vi "WriteVisOptionsToINIFile.vi"(7 "section (optional)":string="Logging and Visualization", 8 "error in (no error)":errorcluster, 10 "Visualization Options":T1={"PauseAtStartup"=TRUE, "LogData"=FALSE, "LaunchInSubPanel"=TRUE, "FPMonitor"=0, "FPWindowBounds"={"Left"=0, "Top"=0, "Right"=0, "Bottom"=0}, "MonitorBounds"={"Left"=0, "Top"=0, "Right"=0, "Bottom"=0}, "MeasIndices"=[]}, 11 "INIFilePath":path) -> (0 "error out":errorcluster, 3 "INI File Path out":path)   [LabVIEW 2018, in "Visualization.lvlib" / "VisualizeBase.lvclass"]
uses:
  VisualizeBase.lvclass
  VisualizationOptions.ctl
  <vilib>/Utility/miscctls.llb/LVRectTypeDef.ctl
  <vilib>/Utility/config.llb/NI_LVConfig.lvlib
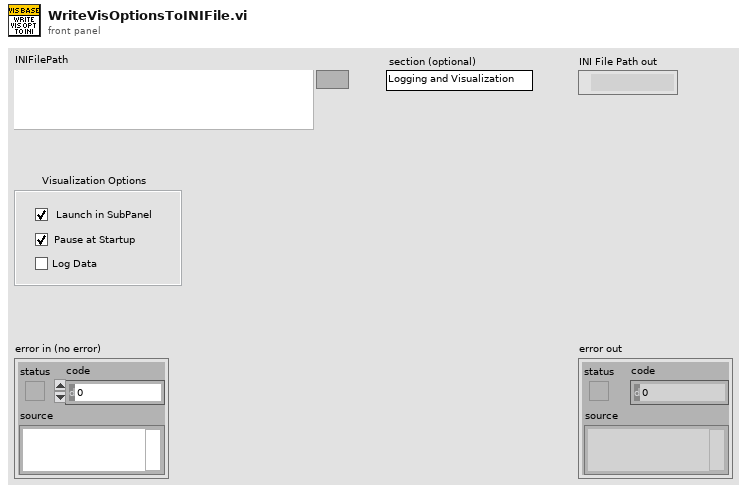
[diagram p1: front panel]
types:
  T1 = typedef "Visualization.lvlib/VisualizeBase.lvclass/VisualizationOptions.ctl" = cluster{"PauseAtStartup":bool, "LogData":bool, "LaunchInSubPanel":bool, "FPMonitor":u16, "FPWindowBounds":T2, "MonitorBounds":cluster{"Left":i16, "Top":i16, "Right":i16, "Bottom":i16}, "MeasIndices":i32[]}
  T2 = typedef "LVRectTypeDef.ctl" = cluster{"Left":i16, "Top":i16, "Right":i16, "Bottom":i16}
  T3 = typedef "LVAllMonitorsDisplayTypeDef.ctl" = cluster{"Bounds":cluster{"Left":i16, "Top":i16, "Right":i16, "Bottom":i16}, "Depth":i16}[]
  T4 = cluster{"Bounds":cluster{"Left":i16, "Top":i16, "Right":i16, "Bottom":i16}, "Depth":i16}
  T5 = cluster{"Left":i16, "Top":i16, "Right":i16, "Bottom":i16}
  T6 = typedef "NI_LVConfig.lvlib/Config Data RefNum.ctl" = refnum<k1>
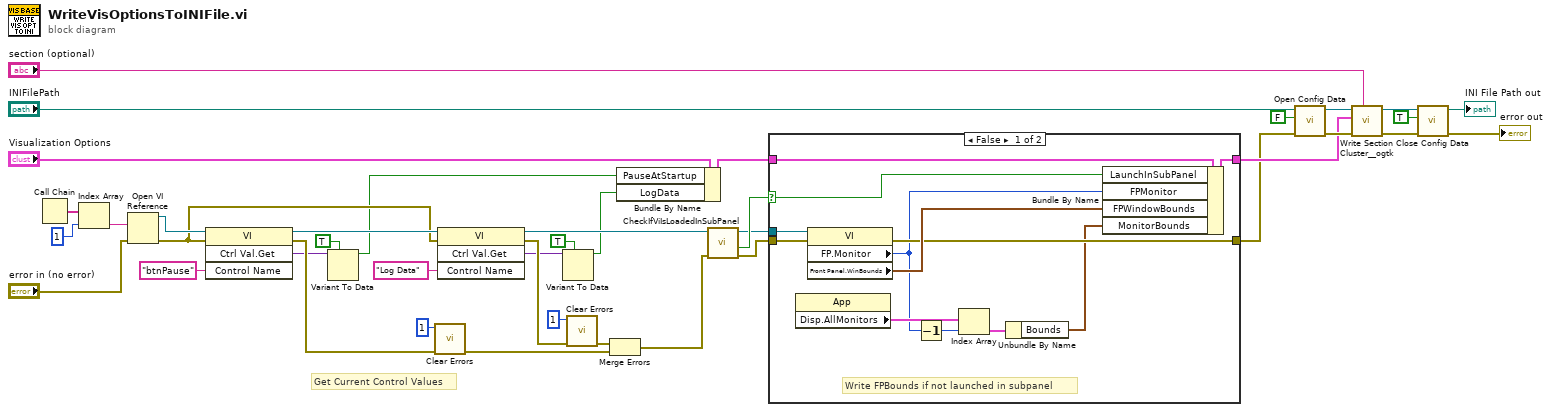
[diagram p0: block diagram]
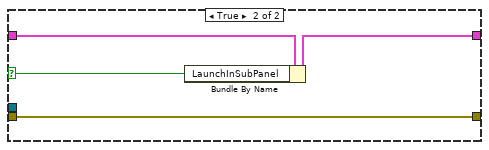
[diagram p2: hidden frame]
diagram:
  # "Get Current Control Values"
  n1 = Call Chain() -> (call chain=w27:string[])
  n2 = Index Array(array=w27, index=1) -> (element=w26:string)
  n3 = Open VI Reference(vi path=w26, error in (no error)="error in (no error)") -> (vi reference=w22:refnum<vi>, error out=w17:errorcluster)  [unwired: 4 in]
  n4 = invoke class="VI" method="Ctrl Val.Get"(reference=w22, error in=w17, "Control Name"="btnPause") -> (reference out=w20:refnum<vi>, error out=w23:errorcluster, "Get Control Value Variant"=w11:variant)  [unwired: 1 in, 1 out]
  n5 = Variant To Data(type=TRUE, Variant=w11) -> (data=w5:bool)  [unwired: 1 in, 1 out]
  n6 = call <vilib>:"Clear Errors.vi"("error in (no error)"=w23, "specific error code to clear (0: all)"=1) -> ("error out"=w12:errorcluster)  [unwired: 4 in, 1 out]
  n7 = invoke class="VI" method="Ctrl Val.Get"(reference=w20, error in=w17, "Control Name"="Log Data") -> (reference out=w19:refnum<vi>, error out=w15:errorcluster, "Get Control Value Variant"=w8:variant)  [unwired: 1 in, 1 out]
  n8 = Variant To Data(type=TRUE, Variant=w8) -> (data=w4:bool)  [unwired: 1 in, 1 out]
  n9 = call <vilib>:"Clear Errors.vi"("error in (no error)"=w15, "specific error code to clear (0: all)"=1) -> ("error out"=w14:errorcluster)  [unwired: 4 in, 1 out]
  n10 = Merge Errors(w14, w12) -> (w13:errorcluster)
  n11 = Bundle By Name(cluster="Visualization Options", "PauseAtStartup"=w5, "LogData"=w4) -> (w7:T1)
  n12 = call "CheckIfViIsLoadedInSubPanel.vi"("error in (no error)"=w13, "vi reference"=w19) -> ("error out"=w3:errorcluster, "In SubPanel?"=w2:bool, "VI reference out"=w1:refnum<vi>)  [unwired: 7 in]
  n13 = case shown="False" w2 {
    selector: w2 -> [w42 w53]
    tunnel: w3 -> [w52 w55]
    tunnel: w7 -> [w51 w56]
    tunnel: [w50 w54] -> w30
    tunnel: [w48 w55] -> w29
    tunnel: w1 -> [w41 _]
    frame False {
      # "Write FPBounds if not launched in subpanel"
      n14 = property class="App"() -> ("Disp.AllMonitors"=w47:T3)  [unwired: 2 in, 2 out]
      n15 = property class="VI"(reference=w41, error in=w52) -> (error out=w48:errorcluster, "FP.Monitor"=w46:u16, "Front Panel.WinBounds"=w49:T2)  [unwired: 1 out]
      n16 = Decrement(x=w46) -> (x-1=w45:u16)
      n17 = Index Array(array=w47, index=w45) -> (element=w44:T4)
      n18 = Unbundle By Name(w44) -> ("Bounds"=w43:T5)
      n19 = Bundle By Name(cluster=w51, "LaunchInSubPanel"=w42, "FPMonitor"=w46, "FPWindowBounds"=w49, "MonitorBounds"=w43) -> (w50:T1)
    }
    frame True {
      n20 = Bundle By Name(cluster=w56, "LaunchInSubPanel"=w53) -> (w54:T1)
    }
  }
  n21 = call <vilib>:"Open Config Data.vi"("error in (no error)"=w29, "create file if necessary (T)"=FALSE, "configuration file path"="INIFilePath") -> ("error out"=w37:errorcluster, "refnum"=w38:T6)  [unwired: 6 in, 1 out]
  n22 = call <userlib>:"Write Section Cluster__ogtk.vi"("section (optional)"="section (optional)", "error in (no error)"=w37, "Section Formatted Cluster"=w30, "refnum"=w38) -> ("error out"=w35:errorcluster, "dup refnum"=w36:T6)  [unwired: 6 in]
  n23 = call <vilib>:"Close Config Data.vi"("error in (no error)"=w35, "write file if changed (T)"=TRUE, "refnum"=w36) -> ("error out"=→"error out":errorcluster, "file path"=→"INI File Path out":path)  [unwired: 7 in]
